vi "Autonomous Independent.vi"() -> ()   [LabVIEW 2013]
doc: "If AutoIDs match then TwoBall? is read from Dashboard, Else it is a control on the Front Panel\n\nINPUTS:\nTwoBall?\nState (Init)\nCollectorArmSpeed\nBrakeDistance\nSlowdownDistance\n\nSTATES:\n\nINIT: Clapper - In, SonicShifter Actuates to Low Gear, RollerPnuematic - Out, Servo - SetAngle (Indicator on Front Panel), IF TwoBall? == True: LowerArm ELSE CheckHotGoal\n\nCHECKHOTGOAL: Runs IsHotGoalDB and puts HotGoal? into Shift Register\n\nLOWERARM: Clapper - OUT, Wait = LowerArmTimeout / 2, RollerPneumatic - WAIT, Collector- LOWER\nWhen Collector has finished or after timeout from LowerArmTimeout and two other timers, Collector - STOP\nIF TwoBall? == TRUE then Collect ELSE Drive12ft\n\nPRECOLLECT: CollectorWrapper - PRECOLLECT\n\nDRIVEBACK: TankDrive -SETVALUE and DriveBackSpeed goes into both desired speeds, Wait - DriveBackWait, TankDrive - SETVALUE and 0 for both desired speeds\n\nCOLLECT: CollectWrapper - COLLECT\n\nSTOPCOLLECT: CollectWrapper - STOP\n\nLIFTARM: Collector - RAISE, Wait - LiftArmWait, Collector - STOP\n\nRAISESERVO: Servo - SETANGLE, Servo takes in RaiseServoAngle from Front Panel\n\nDRIVE12FT: Sonar - READVALUE, AutoDistance - LINEAR, Takes in Drive12ftDistance and distance from the Sonar and BrakeDistance and SlowdownDistance, TankDrive - LINEARDRIVE, Takes in both motor values from AutoDistance and MaxMotorChangeForward/Backward for Desired, TankDrive - LINEARDRIVE, Takes in 0 for Desired and MaxMotorChanges\n\nSHOOT12FT: IF not TwoBall? AND not HotGoal? then Wait - 5500 - ElapsedTime ELSE Pass, Wait - PreShootWait, ShooterWrapper - COLLECTORDOWN\n\nRAISEARM: Wait - PreRaiseArmWait, Collector - RAISE, Takes in CollectorArmSpeed, After Timeout from RaiseArmTimeout or Collector is done , Collector - STOP\n\nSHOOT3FT: Sonar - READVALUE, AutoDistance - LINEAR, Takes in Drive3ftDistance and output form Sonar and Brake/SlowdownDistance, TankDrive - SETVALUE, Takes in AutoDistance values for desired, Exits after AutoDistance is done or Drive3tfTimeout, TankDrive - SETVALUE, Takes in 0 for desired\n\nSHOOT3FT: ShooterWrapper - COLLECTORUP\n\nSTOP: Servo - SETANGLE, 0 for angle"
uses:
  AutoStates.ctl
  AutoMode.ctl
  CollectorAction.ctl
  TankDriveAction.ctl
  CollectorWrapAction.ctl
  ServoAction.ctl
  SonarAction.ctl
  AutoAlignMode.ctl
  ShooterWrapperAction.ctl
  LEDSaction.ctl
  SingleSolenoidAction.ctl
  Robot Global Data.vi
panel:
  in  "Defaults":T1(tab)
  in  "DefaultMotorInput":dbl=1.0
  in  "LowerArmTimeout":u32=800
  in  "PreRaiseArmWait":u32=500
  in  "RaiseArmTimeout":u32=800
  in  "CollectorArmSpeed":dbl=1.0 format="%#_13g"
  in  "PreCollectWait":u32=400
  in  "RotateMotorInput":dbl=0.7
  in  "RotateWait":u32=300
  in  "CheckHotGoalTimeout":u32=800
  out "KinectTriggered?":bool
  out "CheckGoalTimedOut?":bool
  in  "RaiseServoAngle":i32=100
  out "ElapsedTime":u32
  out "StateTime":u32
  out "CurrentState":T2
  out "RaiseArmTimedOut":bool
  out "Hot?":bool
  out "DriveTimeOut":bool
  out "LowerArmTimedOut":bool
  in  "LiftArmWait":u32=200
  in  "PreDriveBackWait":u32
  in  "PreDriveBackSpeed":dbl
  in  "error in":errorcluster
  out "error out":errorcluster
  # "SERVO"
  # "OUTPUT"
  # "DEPRECATED"
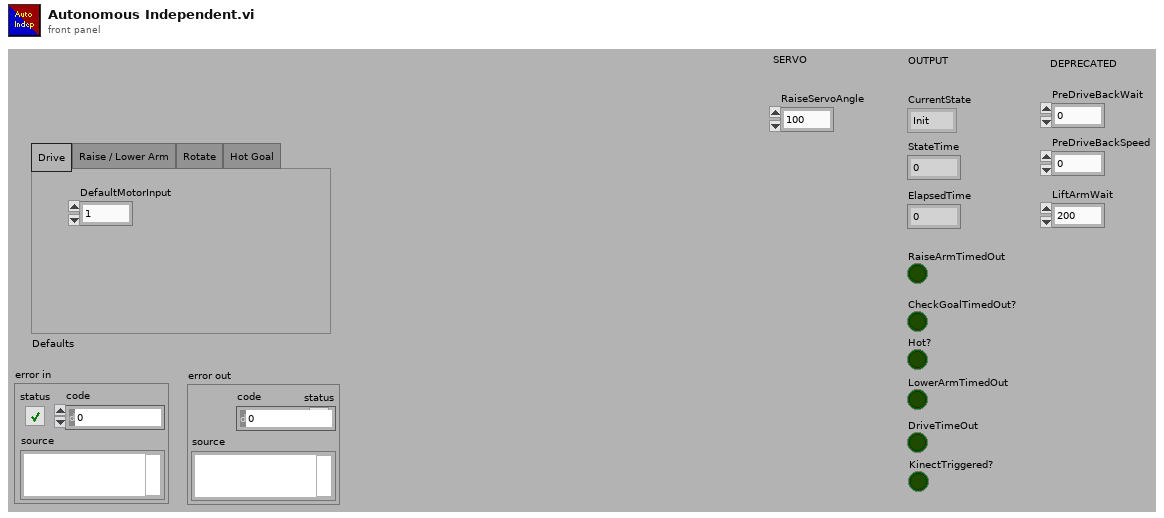
[diagram p1: front panel]
types:
  T1 = enum32{"Drive", "Raise / Lower Arm", "Rotate", "Hot Goal"}
  T2 = typedef "AutoStates.ctl" = enum16{"Init", "LowerArmCheckGoal", "DriveBack", "Collect", "StopCollect", "LiftArm", "RaiseServo", "Drive", "ShootCollectorUp", "RaiseArm", "ShootCollectorDown", "Rotate1", "Rotate2", "Stop"}
  T3 = typedef "AutoData.ctl" = cluster{"StartInLowGear?":bool, "AutoMode":T4, "PreScumbagWait":u32, "DriveTimeout":u32, "DriveMinTime":u32, "DriveDistance":dbl, "StartShootTime":u32, "Brake":dbl, "Slowdown":dbl, "PreCheckGoalWait":u32, "BallSettleWait":u32, "AccelForward":dbl, "AccelBackward":dbl, "HotGoalType":T5, "EndInLowGear?":bool, "DriveBackSpeed":dbl, "DriveBackTime":u32}
  T4 = typedef "AutoMode.ctl" = enum16{"OneBallFront", "OneBallCollector", "TwoBallNormal", "TwoBallHot"}
  T5 = typedef "HotGoalDetectType.ctl" = enum16{"VisionTarget", "Kinect", "SoundDetect", "Webcam"}
  T6 = typedef "CollectorAction.ctl" = enum16{"Init", "Raise", "Lower", "Stop", "GetStatus"}
  T7 = typedef "TankDriveAction.ctl" = enum16{"Init", "LinearDrive", "SetValue", "Disable"}
  T8 = typedef "CollectorWrapAction.ctl" = enum16{"Stop", "PreCollect", "Collect"}
  T9 = typedef "ServoAction.ctl" = enum16{"Init", "SetAngle", "GetAngle", "Lower", "Raise", "Disable"}
  T10 = typedef "AutoAlignMode.ctl" = enum16{"Fullspeed", "Linear"}
  T11 = typedef "SonarAction.ctl" = enum16{"Init", "ReadValue", "Disable"}
  T12 = typedef "LEDSaction.ctl" = enum16{"Init", "10SecondsLeft", "LimitDown", "LimitUp", "CollectDown", "CollectUp", "NotHot", "Hot", "Shift", "RollBack", "RollFwd", "Shoot", "Distance Low", "DistanceHigh", "PressureLow", "PressureHigh"}
  T13 = typedef "ShooterWrapperAction.ctl" = enum16{"Init", "CollectorDown", "CollectorUp"}
  T14 = typedef "SingleSolenoidAction.ctl" = enum16{"Init", "SetState", "Disable"}
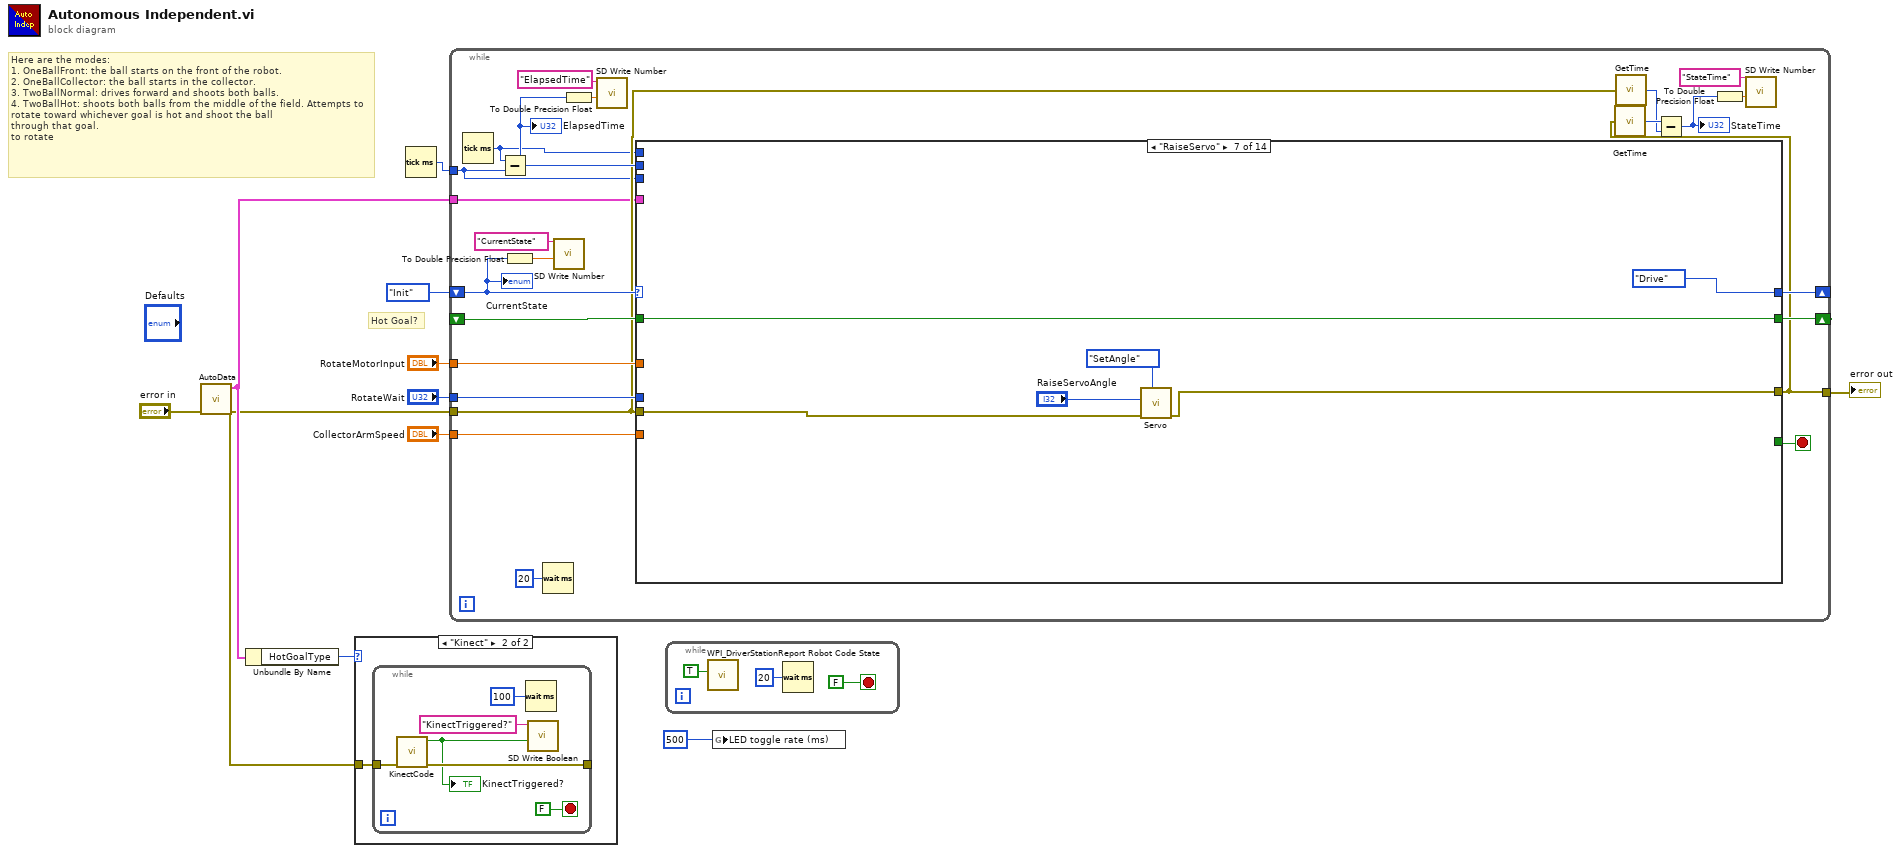
[diagram p0: block diagram]
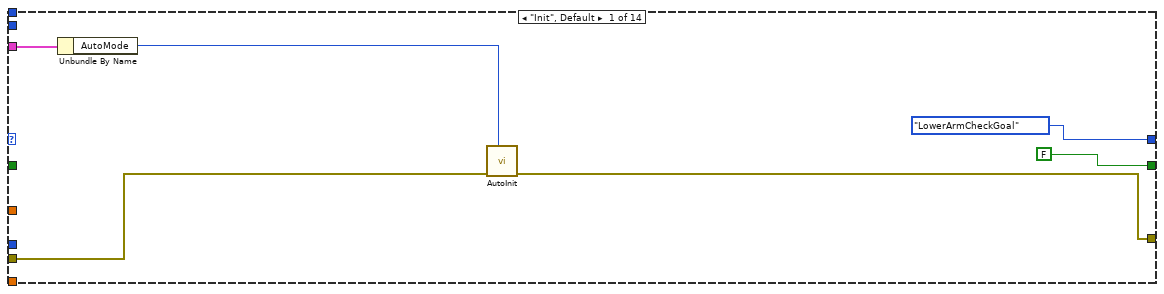
[diagram p3: hidden frame]
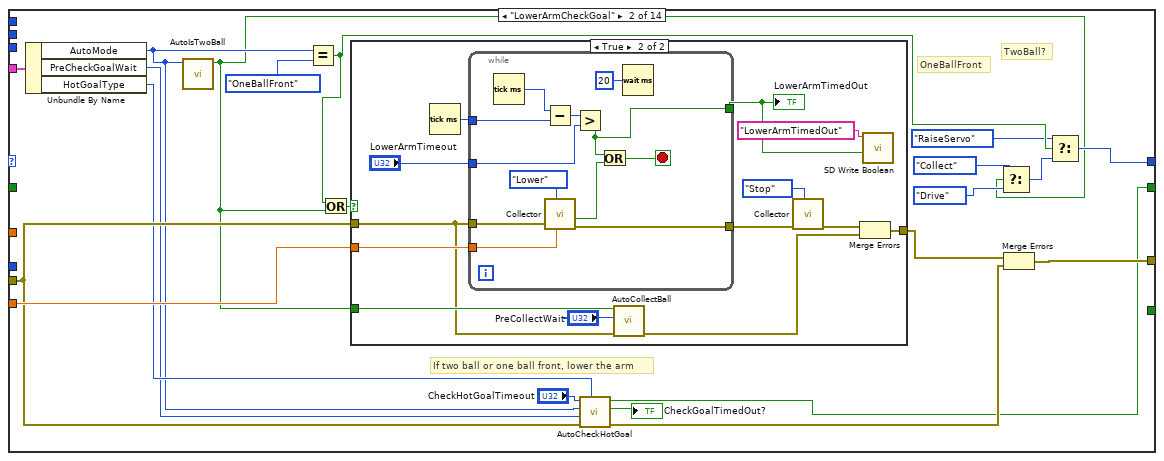
[diagram p4: hidden frame]
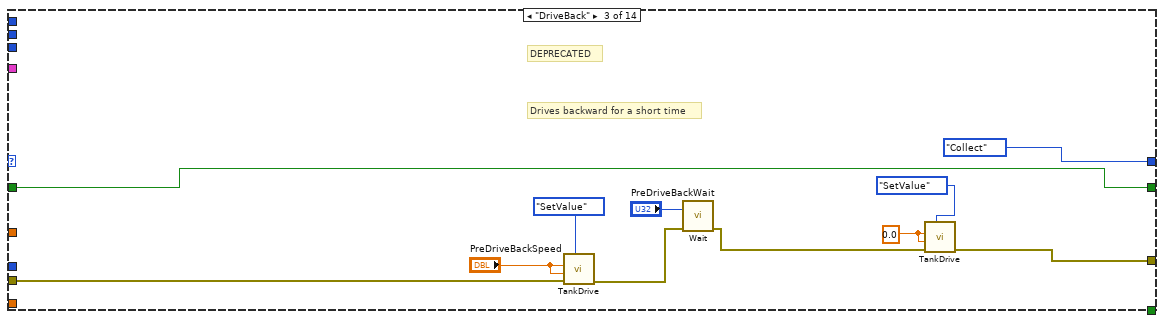
[diagram p6: hidden frame]
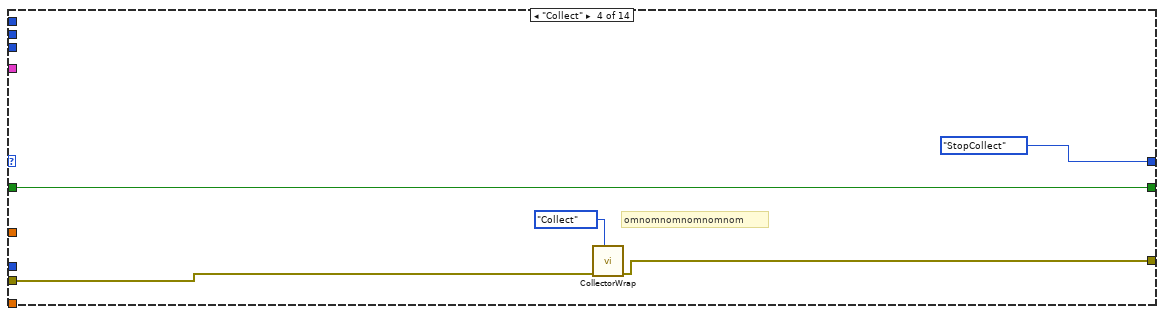
[diagram p7: hidden frame]
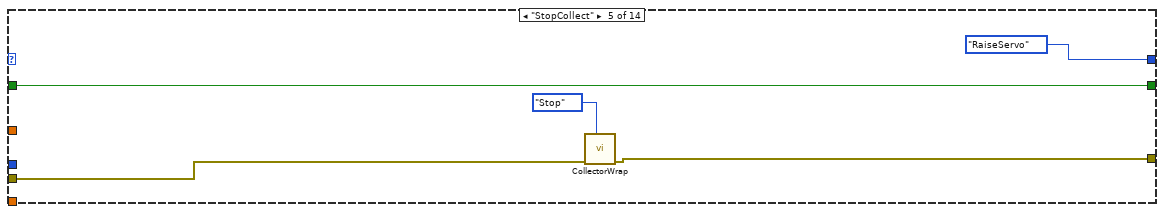
[diagram p8: hidden frame]
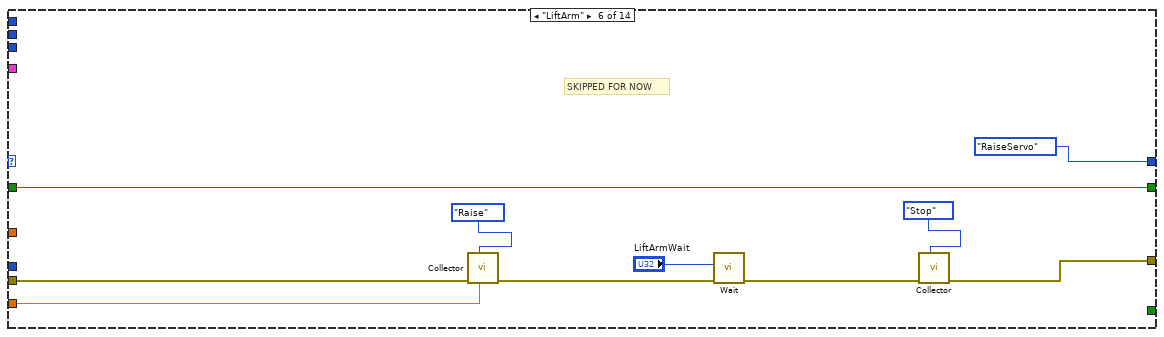
[diagram p9: hidden frame]
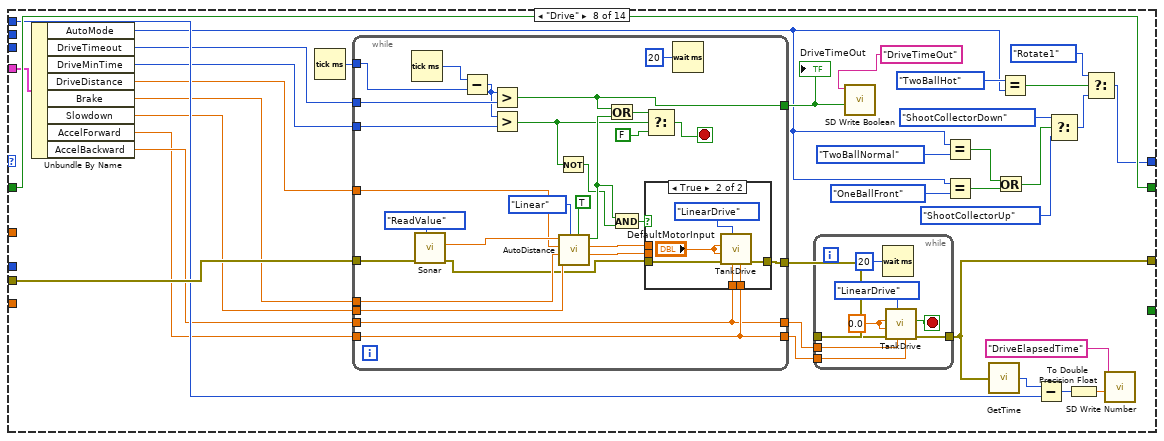
[diagram p10: hidden frame]
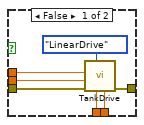
[diagram p11: hidden frame]
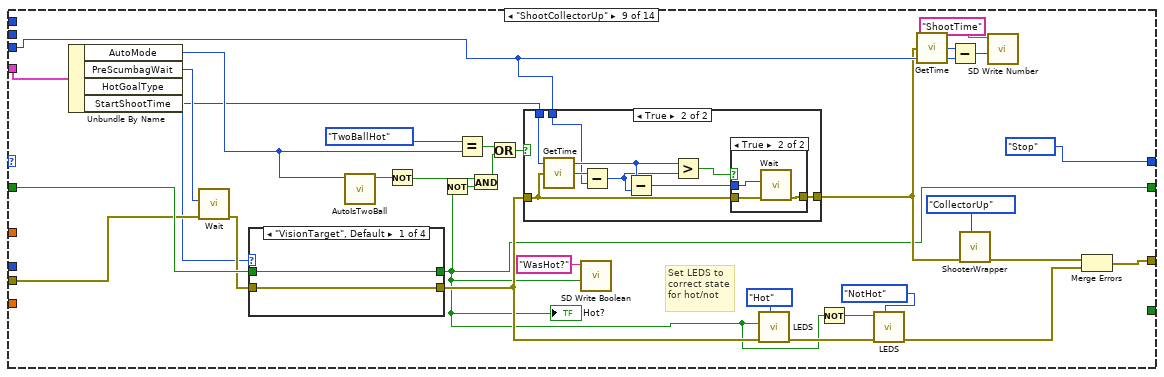
[diagram p12: hidden frame]
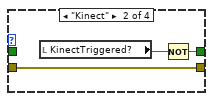
[diagram p13: hidden frame]
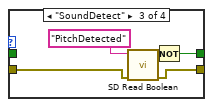
[diagram p14: hidden frame]
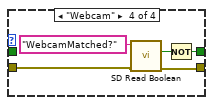
[diagram p15: hidden frame]
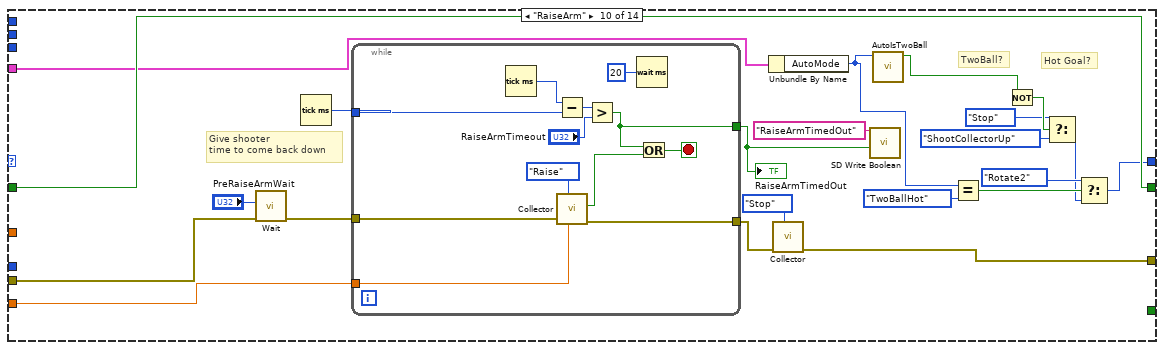
[diagram p18: hidden frame]
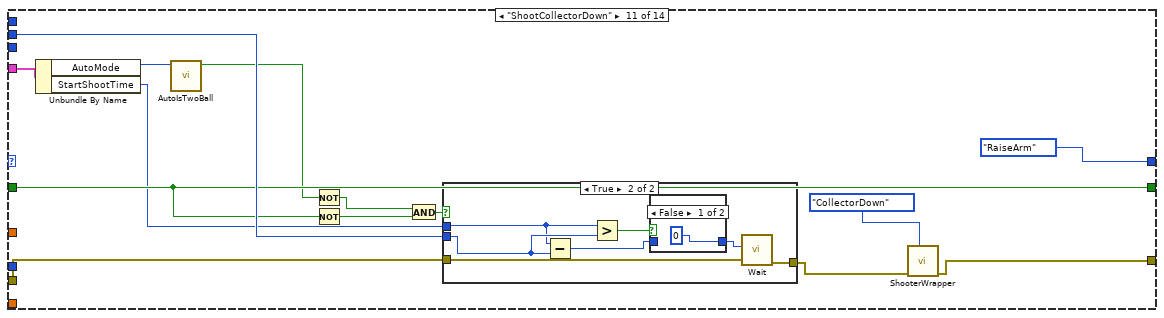
[diagram p19: hidden frame]
diagram:
  # "Here are the modes:\n1. OneBallFront: the ball starts on the front of the robot.\n2. OneBallCollector: the ball starts in the collector.\n3. TwoBallNormal: drives forward and shoots both balls.\n4. TwoBallHot: shoots both balls from the middle of the field. Attempts to rotate toward whichever goal is hot and shoot the ball\nthrough that goal.\nto rotate"
  # "Hot Goal?"
  n1 = call "AutoData.vi"("error in (no error)"="error in") -> ("error out"=w1:errorcluster, "AutoData"=w3:T3)  [unwired: 9 in]
  n2 = Unbundle By Name(w3) -> ("HotGoalType"=w2:T5)
  n3 = case shown="\"Kinect\"" w2 {
    tunnel: w1 -> [_ w12]
    frame "VisionTarget", Default {
    }
    frame "Kinect" {
      n4 = while {
        tunnel: [w16] -> _
        tunnel: w12 -> [w13]
        stop <- FALSE stop-if-true
        n5 = call "KinectCode.vi"("error in"=w13) -> ("error out"=w16:errorcluster, "HandsApart?"=w15:bool)  [unwired: 9 in]
        "KinectTriggered?" <- w15
        n6 = Wait (ms)(milliseconds to wait=u32 100) -> ()  [unwired: 1 out]
        n7 = call <vilib>:"SD Write Boolean.vi"("Boolean"=w15, "Name"="KinectTriggered?") -> ()  [unwired: 8 in, 2 out]
      }
    }
  }
  n8 = Tick Count (ms)() -> (millisecond timer value=w8:u32)
  n9 = while {
    shift-right: [w40] -> _
    shift-left: AutoStates."Init" ("Enum") -> [w26]
    shift-right: [w42] -> _
    shift-left: _ -> [w41]
    tunnel: "CollectorArmSpeed" -> [w38]
    tunnel: w8 -> [w20]
    tunnel: w1 -> [w23]
    tunnel: [w24] -> w11
    tunnel: "RotateMotorInput" -> [w35]
    tunnel: "RotateWait" -> [w34]
    tunnel: w3 -> [w19]
    stop <- w37 stop-if-true
    n10 = Tick Count (ms)() -> (millisecond timer value=w21:u32)
    n11 = Subtract(x=w21, y=w20) -> (x-y=w29:u32)
    "ElapsedTime" <- w29
    n12 = To Double Precision Float(number=w26) -> (double precision float=w27:dbl)
    n13 = Wait (ms)(milliseconds to wait=u32 20) -> ()  [unwired: 1 out]
    n14 = call <vilib>:"SD Write Number.vi"("Numeric"=w27, "Name"="CurrentState") -> ()  [unwired: 8 in, 2 out]
    n15 = To Double Precision Float(number=w29) -> (double precision float=w28:dbl)
    n16 = call <vilib>:"SD Write Number.vi"("Numeric"=w28, "Name"="ElapsedTime") -> ()  [unwired: 8 in, 2 out]
    n17 = case shown="\"RaiseServo\"" w26 {
      selector: w26 -> [_ _ _ _ _ _ _ _ _ _ _ _ _ w393]
      tunnel: w23 -> [w45 w67 w106 w111 w116 w121 w131 w166 w236 w296 w319 w342 w358 w378]
      tunnel: [w46 w66 w99 w110 w115 w120 w130 w134 w231 w294 w324 w337 w357 w381] -> w24
      tunnel: [FALSE ("Hot?") w56 w104 w108 w113 w119 w132 w158 w217 w295 w315 w340 w351 w394] -> w42
      tunnel: w41 -> [_ _ w104 w108 w113 w119 w132 w158 w240 w295 w315 w340 w351 w394]
      tunnel: [AutoStates."LowerArmCheckGoal" ("Enum") w57 AutoStates."Collect" ("Enum") AutoStates."StopCollect" ("Enum") AutoStates."RaiseServo" ("Enum") AutoStates."RaiseServo" ("Enum") AutoStates."Drive" ("Enum") w156 AutoStates."Stop" ("Enum") w282 AutoStates."RaiseArm" ("Enum") AutoStates."ShootCollectorDown" ("Enum") AutoStates."ShootCollectorUp" ("Enum") w393] -> w40
      tunnel: w38 -> [_ w68 _ _ _ w118 _ _ _ w297 _ _ _ _]
      tunnel: w29 -> [_ _ _ _ _ _ _ _ _ _ w317 _ _ _]
      tunnel: [_ _ _ _ _ _ _ _ _ _ _ _ _ TRUE] -> w37
      tunnel: w35 -> [_ _ _ _ _ _ _ _ _ _ _ w347 w360 _]
      tunnel: w34 -> [_ _ _ _ _ _ _ _ _ _ _ w339 w359 _]
      tunnel: w21 -> [_ _ _ _ _ _ _ w147 _ _ _ _ _ _]
      tunnel: w20 -> [_ _ _ _ _ _ _ _ w234 _ _ _ _ _]
      tunnel: w19 -> [w43 w55 _ _ _ _ _ w145 w230 w279 w314 _ _ w372]
      frame "Init", Default {
        n18 = Unbundle By Name(w43) -> ("AutoMode"=w44:T4)
        n19 = call "AutoInit.vi"("AutoMode"=w44, "error in (no error)"=w45) -> ("error out"=w46:errorcluster)  [unwired: 9 in]
      }
      frame "LowerArmCheckGoal" {
        # "If two ball or one ball front, lower the arm"
        # "OneBallFront"
        # "TwoBall?"
        n20 = Unbundle By Name(w55) -> ("AutoMode"=w52:T4, "PreCheckGoalWait"=w53:u32, "HotGoalType"=w54:T5)
        n21 = call "AutoIsTwoBall.vi"("AutoMode"=w52) -> ("IsTwoBall?"=w51:bool)  [unwired: 10 in]
        n22 = Equal?(x=w52, y=AutoMode."OneBallFront") -> (x = y?=w60:bool)
        n23 = Or(x=w60, y=w51) -> (x .or. y?=w63:bool)
        n24 = case shown="True" w63 {
          tunnel: w68 -> [_ w82]
          tunnel: [w70 w71] -> w61
          tunnel: w67 -> [w70 w77]
          tunnel: w51 -> [_ w78]
          frame False {
          }
          frame True {
            n25 = Tick Count (ms)() -> (millisecond timer value=w83:u32)
            n26 = while {
              tunnel: w77 -> [w84]
              tunnel: [w95] -> w79
              tunnel: w83 -> [w88]
              tunnel: w82 -> [w87]
              tunnel: [w86] -> w76
              tunnel: "LowerArmTimeout" -> [w85]
              stop <- w90 stop-if-true
              n27 = Tick Count (ms)() -> (millisecond timer value=w92:u32)
              n28 = Subtract(x=w92, y=w88) -> (x-y=w93:u32)
              n29 = call "Collector.vi"("MotorSpeed"=w87, "Action"=CollectorAction."Lower", "Error in"=w84) -> ("Error out"=w95:errorcluster, "Lower Triggered?"=w89:bool)  [unwired: 6 in, 1 out]
              n30 = Greater?(x=w93, y=w85) -> (0:w86:bool)
              n31 = Or(x=w86, y=w89) -> (x .or. y?=w90:bool)
              n32 = Wait (ms)(milliseconds to wait=u32 20) -> ()  [unwired: 1 out]
            }
            "LowerArmTimedOut" <- w76
            n33 = call "AutoCollectBall.vi"("error in (no error)"=w77, "PreCollectWait"="PreCollectWait", "IsTwoBall?"=w78) -> ("error out"=w73:errorcluster)  [unwired: 8 in]
            n34 = call "Collector.vi"("Action"=CollectorAction."Stop", "Error in"=w79) -> ("Error out"=w72:errorcluster)  [unwired: 7 in, 2 out]
            n35 = Merge Errors(w72, w73) -> (w71:errorcluster)
            n36 = call <vilib>:"SD Write Boolean.vi"("Boolean"=w76, "Name"="LowerArmTimedOut") -> ()  [unwired: 8 in, 2 out]
          }
        }
        n37 = call "AutoCheckHotGoal.vi"("HotGoalType"=w54, "error in (no error)"=w67, "PreCheckGoalWait"=w53, "AutoMode"=w52, "CheckHotGoalTimeout"="CheckHotGoalTimeout") -> ("error out"=w65:errorcluster, "CheckGoalTimedOut?"=→"CheckGoalTimedOut?":bool, "Hot?"=w56:bool)  [unwired: 4 in]
        n38 = Select(t=AutoStates."Collect" ("Enum"), s=w51, f=AutoStates."Drive" ("Enum")) -> (s? t:f=w58:T2)
        n39 = Merge Errors(w61, w65) -> (w66:errorcluster)
        n40 = Select(t=AutoStates."RaiseServo" ("Enum"), s=w60, f=w58) -> (s? t:f=w57:T2)
      }
      frame "DriveBack" {
        w97 = 0.0 ("LeftDesired")
        # "Drives backward for a short time"
        # "DEPRECATED"
        n41 = call "TankDrive.vi"("DriveAction"=TankDriveAction."SetValue", "error in (no error)"=w106, "RightDesired"="PreDriveBackSpeed", "LeftDesired"="PreDriveBackSpeed") -> ("error out"=w105:errorcluster)  [unwired: 6 in, 1 out]
        n42 = call "Wait.vi"("error in"=w105, "milliseconds to wait"="PreDriveBackWait") -> ("error out"=w100:errorcluster)  [unwired: 9 in]
        n43 = call "TankDrive.vi"("DriveAction"=TankDriveAction."SetValue", "error in (no error)"=w100, "RightDesired"=w97, "LeftDesired"=w97) -> ("error out"=w99:errorcluster)  [unwired: 6 in, 1 out]
      }
      frame "Collect" {
        # "omnomnomnomnomnom"
        n44 = call "CollectorWrap.vi"("Action"=CollectorWrapAction."Collect", "error in"=w111) -> ("error out"=w110:errorcluster)  [unwired: 9 in]
      }
      frame "StopCollect" {
        n45 = call "CollectorWrap.vi"("Action"=CollectorWrapAction."Stop", "error in"=w116) -> ("error out"=w115:errorcluster)  [unwired: 9 in]
      }
      frame "LiftArm" {
        # "SKIPPED FOR NOW"
        n46 = call "Collector.vi"("MotorSpeed"=w118, "Action"=CollectorAction."Raise" ("CollectorAction"), "Error in"=w121) -> ("Error out"=w122:errorcluster)  [unwired: 6 in, 2 out]
        n47 = call "Wait.vi"("error in"=w122, "milliseconds to wait"="LiftArmWait") -> ("error out"=w123:errorcluster)  [unwired: 9 in]
        n48 = call "Collector.vi"("Action"=CollectorAction."Stop" ("CollectorAction"), "Error in"=w123) -> ("Error out"=w120:errorcluster)  [unwired: 7 in, 2 out]
      }
      frame "RaiseServo" {
        n49 = call "Servo.vi"("Action"=ServoAction."SetAngle", "error in (no error)"=w131, "Angle (deg)"="RaiseServoAngle") -> ("error out"=w130:errorcluster)  [unwired: 7 in, 1 out]
      }
      frame "Drive" {
        n50 = Unbundle By Name(w145) -> ("AutoMode"=w144:T4, "DriveTimeout"=w143:u32, "DriveMinTime"=w142:u32, "DriveDistance"=w141:dbl, "Brake"=w140:dbl, "Slowdown"=w139:dbl, "AccelForward"=w137:dbl, "AccelBackward"=w138:dbl)
        n51 = Tick Count (ms)() -> (millisecond timer value=w167:u32)
        n52 = while {
          tunnel: w166 -> [w196]
          tunnel: [w200] -> w152
          tunnel: w167 -> [w201]
          tunnel: w139 -> [w198]
          tunnel: w140 -> [w199]
          tunnel: [w185] -> w151
          tunnel: w137 -> [w177]
          tunnel: w138 -> [w176]
          tunnel: w143 -> [w192]
          tunnel: w141 -> [w191]
          tunnel: w142 -> [w186]
          tunnel: [w177] -> w136
          tunnel: [w176] -> w135
          stop <- w183 stop-if-true
          n53 = Tick Count (ms)() -> (millisecond timer value=w202:u32)
          n54 = call "Sonar.vi"("Action"=SonarAction."ReadValue", "error in (no error)"=w196) -> ("error out"=w193:errorcluster, "distance"=w195:dbl)  [unwired: 8 in]
          n55 = Subtract(x=w202, y=w201) -> (x-y=w187:u32)
          n56 = Greater?(x=w187, y=w192) -> (0:w185:bool)
          n57 = Greater?(x=w187, y=w186) -> (0:w180:bool)
          n58 = Not(x=w180) -> (.not. x?=w179:bool)
          n59 = call "AutoDistance.vi"("Auto"=TRUE, "Mode"=AutoAlignMode."Linear", "Slowdown"=w198, "Brake"=w199, "DesiredDistance"=w191, "CurrentDistance"=w195) -> ("TankDriveRight"=w189:dbl, "TankDriveLeft"=w188:dbl, "Finished"=w181:bool)  [unwired: 3 in]
          n60 = Or(x=w185, y=w181) -> (x .or. y?=w184:bool)
          n61 = And(x=w181, y=w179) -> (x .and. y?=w182:bool)
          n62 = case shown="True" w182 {
            tunnel: [w209 w215] -> w200
            tunnel: w193 -> [w208 w214]
            tunnel: w177 -> [w204 w213]
            tunnel: w176 -> [w205 w212]
            tunnel: w189 -> [w206 _]
            tunnel: w188 -> [w207 _]
            frame False {
              n63 = call "TankDrive.vi"("MaxMotorChangeForward"=w204, "MaxMotorChangeBackwrad"=w205, "DriveAction"=TankDriveAction."LinearDrive", "error in (no error)"=w208, "RightDesired"=w206, "LeftDesired"=w207) -> ("error out"=w209:errorcluster)  [unwired: 4 in, 1 out]
            }
            frame True {
              n64 = call "TankDrive.vi"("MaxMotorChangeForward"=w213, "MaxMotorChangeBackwrad"=w212, "DriveAction"=TankDriveAction."LinearDrive", "error in (no error)"=w214, "RightDesired"="DefaultMotorInput", "LeftDesired"="DefaultMotorInput") -> ("error out"=w215:errorcluster)  [unwired: 4 in, 1 out]
            }
          }
          n65 = Select(t=w184, s=w180, f=FALSE) -> (s? t:f=w183:bool)
          n66 = Wait (ms)(milliseconds to wait=u32 20) -> ()  [unwired: 1 out]
        }
        "DriveTimeOut" <- w151
        n67 = while {
          tunnel: w152 -> [w175]
          tunnel: [w168] -> w134
          tunnel: w136 -> [w170]
          tunnel: w135 -> [w169]
          stop <- w171 stop-if-true
          w174 = 0.0 ("LeftDesired")
          n68 = Wait (ms)(milliseconds to wait=u32 20) -> ()  [unwired: 1 out]
          n69 = call "TankDrive.vi"("MaxMotorChangeForward"=w170, "MaxMotorChangeBackwrad"=w169, "DriveAction"=TankDriveAction."LinearDrive", "error in (no error)"=w175, "RightDesired"=w174, "LeftDesired"=w174) -> ("error out"=w168:errorcluster, "InRange?"=w171:bool)  [unwired: 4 in]
        }
        n70 = call <vilib>:"SD Write Boolean.vi"("Boolean"=w151, "Name"="DriveTimeOut") -> ()  [unwired: 8 in, 2 out]
        n71 = Equal?(x=w144, y=AutoMode."TwoBallNormal") -> (x = y?=w164:bool)
        n72 = Equal?(x=w144, y=AutoMode."OneBallFront") -> (x = y?=w163:bool)
        n73 = call "GetTime.vi"("error in"=w134) -> ("Time"=w133:u32)
        n74 = Or(x=w164, y=w163) -> (x .or. y?=w159:bool)
        n75 = Equal?(x=AutoMode."TwoBallHot" ("y"), y=w144) -> (x = y?=w154:bool)
        n76 = Subtract(x=w133, y=w147) -> (x-y=w148:u32)
        n77 = Select(t=AutoStates."ShootCollectorDown" ("Enum"), s=w159, f=AutoStates."ShootCollectorUp") -> (s? t:f=w157:T2)
        n78 = To Double Precision Float(number=w148) -> (double precision float=w149:dbl)
        n79 = Select(t=AutoStates."Rotate1" ("Enum"), s=w154, f=w157) -> (s? t:f=w156:T2)
        n80 = call <vilib>:"SD Write Number.vi"("Numeric"=w149, "Name"="DriveElapsedTime") -> ()  [unwired: 8 in, 2 out]
      }
      frame "ShootCollectorUp" {
        # "Set LEDS to\ncorrect state\nfor hot/not"
        n81 = Unbundle By Name(w230) -> ("AutoMode"=w228:T4, "PreScumbagWait"=w229:u32, "HotGoalType"=w226:T5, "StartShootTime"=w225:u32)
        n82 = call "Wait.vi"("error in"=w236, "milliseconds to wait"=w229) -> ("error out"=w235:errorcluster)  [unwired: 9 in]
        n83 = case shown="\"VisionTarget\", Default" w226 {
          tunnel: w240 -> [w250 _ _ _]
          tunnel: [w250 w252 w256 w261] -> w217
          tunnel: w235 -> [w249 w251 w255 w260]
          tunnel: [w249 w251 w254 w259] -> w218
          frame "VisionTarget", Default {
          }
          frame "Kinect" {
            n84 = local read "KinectTriggered?"() -> (w253:bool)
            n85 = Not(x=w253) -> (.not. x?=w252:bool)
          }
          frame "SoundDetect" {
            n86 = call <vilib>:"SD Read Boolean.vi"("error in"=w255, "Name"="PitchDetected") -> ("error out"=w254:errorcluster, "Boolean"=w258:bool)  [unwired: 7 in, 1 out]
            n87 = Not(x=w258) -> (.not. x?=w256:bool)
          }
          frame "Webcam" {
            n88 = call <vilib>:"SD Read Boolean.vi"("error in"=w260, "Name"="WebcamMatched?") -> ("error out"=w259:errorcluster, "Boolean"=w263:bool)  [unwired: 7 in, 1 out]
            n89 = Not(x=w263) -> (.not. x?=w261:bool)
          }
        }
        "Hot?" <- w217
        n90 = call "AutoIsTwoBall.vi"("AutoMode"=w228) -> ("IsTwoBall?"=w227:bool)  [unwired: 10 in]
        n91 = Not(x=w227) -> (.not. x?=w247:bool)
        n92 = Not(x=w217) -> (.not. x?=w246:bool)
        n93 = Equal?(x=AutoMode."TwoBallHot" ("y"), y=w228) -> (x = y?=w242:bool)
        n94 = And(x=w247, y=w246) -> (x .and. y?=w244:bool)
        n95 = Or(x=w242, y=w244) -> (x .or. y?=w243:bool)
        n96 = case shown="True" w243 {
          tunnel: w218 -> [w264 w266]
          tunnel: [w264 w265] -> w223
          tunnel: w225 -> [_ w270]
          tunnel: w234 -> [_ w268]
          frame False {
          }
          frame True {
            n97 = call "GetTime.vi"("error in"=w266) -> ("Time"=w269:u32)
            n98 = Subtract(x=w269, y=w268) -> (x-y=w267:u32)
            n99 = Subtract(x=w270, y=w267) -> (x-y=w271:u32)
            n100 = Greater?(x=w270, y=w267) -> (0:w272:bool)
            n101 = case shown="True" w272 {
              tunnel: w271 -> [_ w276]
              tunnel: w266 -> [w273 w275]
              tunnel: [w273 w274] -> w265
              frame False {
              }
              frame True {
                n102 = call "Wait.vi"("error in"=w275, "milliseconds to wait"=w276) -> ("error out"=w274:errorcluster)  [unwired: 9 in]
              }
            }
          }
        }
        n103 = call <vilib>:"SD Write Boolean.vi"("Boolean"=w217, "Name"="WasHot?") -> ()  [unwired: 8 in, 2 out]
        n104 = call "LEDS.vi"("Action"=LEDSaction."Hot", "error in"=w218, "On/Off"=w217) -> ("error out"=w222:errorcluster)  [unwired: 8 in]
        n105 = Not(x=w217) -> (.not. x?=w221:bool)
        n106 = call "LEDS.vi"("Action"=LEDSaction."NotHot", "error in"=w222, "On/Off"=w221) -> ("error out"=w219:errorcluster)  [unwired: 8 in]
        n107 = call "GetTime.vi"("error in"=w223) -> ("Time"=w224:u32)
        n108 = Subtract(x=w224, y=w234) -> (x-y=w237:u32)
        n109 = call "ShooterWrapper.vi"("Action"=ShooterWrapperAction."CollectorUp", "error in"=w223) -> ("error out"=w232:errorcluster)  [unwired: 8 in]
        n110 = call <vilib>:"SD Write Number.vi"("Numeric"=w237, "Name"="ShootTime") -> ()  [unwired: 8 in, 2 out]
        n111 = Merge Errors(w232, w219) -> (w231:errorcluster)
      }
      frame "RaiseArm" {
        # "Hot Goal?"
        # "TwoBall?"
        # "Give shooter\ntime to come back down"
        n112 = call "Wait.vi"("error in"=w296, "milliseconds to wait"="PreRaiseArmWait") -> ("error out"=w292:errorcluster)  [unwired: 9 in]
        n113 = Tick Count (ms)() -> (millisecond timer value=w298:u32)
        n114 = while {
          tunnel: w292 -> [w310]
          tunnel: [w309] -> w290
          tunnel: w298 -> [w302]
          tunnel: w297 -> [w301]
          tunnel: [w300] -> w281
          stop <- w303 stop-if-true
          n115 = Tick Count (ms)() -> (millisecond timer value=w305:u32)
          n116 = Subtract(x=w305, y=w302) -> (x-y=w306:u32)
          n117 = call "Collector.vi"("MotorSpeed"=w301, "Action"=CollectorAction."Raise", "Error in"=w310) -> ("Error out"=w309:errorcluster, "Upper Triggered?"=w299:bool)  [unwired: 6 in, 1 out]
          n118 = Greater?(x=w306, y="RaiseArmTimeout") -> (0:w300:bool)
          n119 = Wait (ms)(milliseconds to wait=u32 20) -> ()  [unwired: 1 out]
          n120 = Or(x=w300, y=w299) -> (x .or. y?=w303:bool)
        }
        "RaiseArmTimedOut" <- w281
        n121 = Unbundle By Name(w279) -> ("AutoMode"=w278:T4)
        n122 = call "Collector.vi"("Action"=CollectorAction."Stop", "Error in"=w290) -> ("Error out"=w294:errorcluster)  [unwired: 7 in, 2 out]
        n123 = call <vilib>:"SD Write Boolean.vi"("Boolean"=w281, "Name"="RaiseArmTimedOut") -> ()  [unwired: 8 in, 2 out]
        n124 = call "AutoIsTwoBall.vi"("AutoMode"=w278) -> ("IsTwoBall?"=w277:bool)  [unwired: 10 in]
        n125 = Equal?(x=w278, y=AutoMode."TwoBallHot") -> (x = y?=w285:bool)
        n126 = Not(x=w277) -> (.not. x?=w289:bool)
        n127 = Select(t=AutoStates."Stop" ("Enum"), s=w289, f=AutoStates."ShootCollectorUp" ("Enum")) -> (s? t:f=w283:T2)
        n128 = Select(t=AutoStates."Rotate2" ("Enum"), s=w285, f=w283) -> (s? t:f=w282:T2)
      }
      frame "ShootCollectorDown" {
        n129 = Unbundle By Name(w314) -> ("AutoMode"=w313:T4, "StartShootTime"=w311:u32)
        n130 = call "AutoIsTwoBall.vi"("AutoMode"=w313) -> ("IsTwoBall?"=w312:bool)  [unwired: 10 in]
        n131 = Not(x=w312) -> (.not. x?=w321:bool)
        n132 = Not(x=w315) -> (.not. x?=w320:bool)
        n133 = And(x=w321, y=w320) -> (x .and. y?=w316:bool)
        n134 = case shown="True" w316 {
          tunnel: w319 -> [w325 w332]
          tunnel: [w325 w331] -> w318
          tunnel: w317 -> [_ w330]
          tunnel: w311 -> [_ w326]
          frame False {
          }
          frame True {
            n135 = Subtract(x=w326, y=w330) -> (x-y=w327:u32)
            n136 = Greater?(x=w326, y=w330) -> (0:w329:bool)
            n137 = case shown="False" w329 {
              tunnel: [u32 0 w334] -> w328
              tunnel: w327 -> [_ w334]
              frame False {
              }
              frame True {
              }
            }
            n138 = call "Wait.vi"("error in"=w332, "milliseconds to wait"=w328) -> ("error out"=w331:errorcluster)  [unwired: 9 in]
          }
        }
        n139 = call "ShooterWrapper.vi"("Action"=ShooterWrapperAction."CollectorDown", "error in"=w318) -> ("error out"=w324:errorcluster)  [unwired: 8 in]
      }
      frame "Rotate1" {
        w336 = 0.0
        # "ASSUME CAMERA POINTED LEFT"
        n140 = Select(t=1.0, s=w340, f=-1.0) -> (s? t:f=w349:dbl)
        n141 = Multiply(x=w349, y=w347) -> (x*y=w346:dbl)
        n142 = Negate(x=w346) -> (-x=w345:dbl)
        n143 = call "TankDrive.vi"("DriveAction"=TankDriveAction."SetValue", "error in (no error)"=w342, "RightDesired"=w346, "LeftDesired"=w345) -> ("error out"=w341:errorcluster)  [unwired: 6 in, 1 out]
        n144 = call "Wait.vi"("error in"=w341, "milliseconds to wait"=w339) -> ("error out"=w338:errorcluster)  [unwired: 9 in]
        n145 = call "TankDrive.vi"("DriveAction"=TankDriveAction."SetValue", "error in (no error)"=w338, "RightDesired"=w336, "LeftDesired"=w336) -> ("error out"=w337:errorcluster)  [unwired: 6 in, 1 out]
      }
      frame "Rotate2" {
        w362 = 0.0
        n146 = Select(t=1.0, s=w351, f=-1.0) -> (s? t:f=w367:dbl)
        n147 = Multiply(x=w367, y=w360) -> (x*y=w356:dbl)
        n148 = Negate(x=w356) -> (-x=w355:dbl)
        n149 = call "TankDrive.vi"("DriveAction"=TankDriveAction."SetValue", "error in (no error)"=w358, "RightDesired"=w355, "LeftDesired"=w356) -> ("error out"=w364:errorcluster)  [unwired: 6 in, 1 out]
        n150 = Multiply(x=u32 2, y=w359) -> (x*y=w354:u32)
        n151 = call "Wait.vi"("error in"=w364, "milliseconds to wait"=w354) -> ("error out"=w363:errorcluster)  [unwired: 9 in]
        n152 = call "TankDrive.vi"("DriveAction"=TankDriveAction."SetValue", "error in (no error)"=w363, "RightDesired"=w362, "LeftDesired"=w362) -> ("error out"=w357:errorcluster)  [unwired: 6 in, 1 out]
      }
      frame "Stop" {
        w385 = 0.0 ("LeftDesired")
        # "Turn off hot/not hot\nLEDs"
        n153 = Unbundle By Name(w372) -> ("EndInLowGear?"=w371:bool, "DriveBackSpeed"=w370:dbl, "DriveBackTime"=w369:u32)
        n154 = call "LEDS.vi"("Action"=LEDSaction."Hot", "error in"=w378, "On/Off"=FALSE) -> ("error out"=w375:errorcluster)  [unwired: 8 in]
        n155 = call "LEDS.vi"("Action"=LEDSaction."NotHot", "error in"=w378, "On/Off"=FALSE) -> ("error out"=w374:errorcluster)  [unwired: 8 in]
        n156 = Merge Errors(w375, w374) -> (w373:errorcluster)
        n157 = call "Servo.vi"("Action"=ServoAction."SetAngle", "error in (no error)"=w373, "Angle (deg)"=0) -> ("error out"=w383:errorcluster)  [unwired: 7 in, 1 out]
        n158 = call "SonicShifter.vi"("Action"=SingleSolenoidAction."SetState", "error in (no error)"=w383, "Actuate?"=w371) -> ("error out"=w382:errorcluster)  [unwired: 8 in]
        n159 = call "TankDrive.vi"("DriveAction"=TankDriveAction."SetValue", "error in (no error)"=w382, "RightDesired"=w370, "LeftDesired"=w370) -> ("error out"=w387:errorcluster)  [unwired: 6 in, 1 out]
        n160 = call "Wait.vi"("error in"=w387, "milliseconds to wait"=w369) -> ("error out"=w386:errorcluster)  [unwired: 9 in]
        n161 = call "TankDrive.vi"("DriveAction"=TankDriveAction."SetValue", "error in (no error)"=w386, "RightDesired"=w385, "LeftDesired"=w385) -> ("error out"=w381:errorcluster)  [unwired: 6 in, 1 out]
      }
    }
    n162 = call "GetTime.vi"("error in"=w24) -> ("Time"=w36:u32)
    n163 = call "GetTime.vi"("error in"=w23) -> ("Time"=w22:u32)
    n164 = Subtract(x=w36, y=w22) -> (x-y=w33:u32)
    "StateTime" <- w33
    n165 = To Double Precision Float(number=w33) -> (double precision float=w31:dbl)
    n166 = call <vilib>:"SD Write Number.vi"("Numeric"=w31, "Name"="StateTime") -> ()  [unwired: 8 in, 2 out]
    "CurrentState" <- w26
  }
  "error out" <- w11
  n167 = while {
    stop <- FALSE stop-if-true
    n168 = call <vilib>:"WPI_DriverStationReport Robot Code State.vi"("Autonomous"=TRUE) -> ()  [unwired: 10 in, 1 out]
    n169 = Wait (ms)(milliseconds to wait=u32 20) -> ()  [unwired: 1 out]
  }
  n170 = global write "Robot Global Data.vi" "LED toggle rate (ms)"(u32 500 ("LED ms toggle rate")) -> ()
